vi "Get_camera_properties.vi"() -> ()   [LabVIEW 2012]
panel:
  in  "Camera Index":u32
  out "Function List":T1(array[cluster])
  out "error out":errorcluster
  out "Parameter Range":cluster{"min":dbl, "max":dbl, "step":dbl}
  out "Default parameter value":dbl
  out "Value Names":cluster{"Name":string, "Value":dbl}[](array[cluster])
  out "Parameter value":dbl
  in  "Parameter to query":u32(ring)=37 items=["BINNING"=1, "BITS PER CHANNEL"=2, "ACTIVE VIEW INDEX"=3, "CCD MODE"=4, "SENSOR MODE"=5, "READOUT MODE"=6, "EXPOSURE TIME"=7, "CONTRAST GAIN"=8, "CONTRAST OFFSET"=9, "LIGHT MODE"=10, "SENSITIVITY"=11, "WHITE BALANCE"=12, "PHOTON IMAGING MODE"=13, "HIGH DYNAMIC RANGE MODE"=14, "TRIGGER SOURCE"=15, "TRIGGER ACTIVE"=16, "TRIGGER MODE"=17, "TRIGGER POLARITY"=18, "TRIGGER GLOBAL EXPOSURE"=19, "FIRST TRIGGER BEHAVIOR"=20, "TRIGGER TIMES"=21, "OUTPUT TRIGGER POLARITY"=22, "OUTPUT TRIGGER DELAY"=23, "OUTPUT TRIGGER PERIOD"=24, "TEMPERATURE"=25, "TEMPERATURE TARGET"=26, "SENSOR COOLER FAN"=27, "MECHANICAL SHUTTER"=28, "BACK FOCUS POSITION"=29, "FRAMEBUNDLE MODE"=30, "FRAMEBUNDLE NUMBER"=31, "LINEBUNDLE HEIGHT"=32, "TRIGGER CONNECTOR"=33, "IMAGE PIXEL TYPE"=34, "OUTPUT TRIGGER KIND"=35, "READOUT DIRECTION"=36]
  out "Camera info":string
  in  "Info ID":u32(ring)=67109121 items=["BUS"=67109121, "CAMERA ID"=67109122, "VENDOR"=67109123, "MODEL"=67109124, "CAMERA VERSION"=67109125, "DRIVER VERSION"=67109126, "MODULE VERSIOIN"=67109127, "DCAMAPI VERSION"=67109128]
  in  "error in (no error)":errorcluster
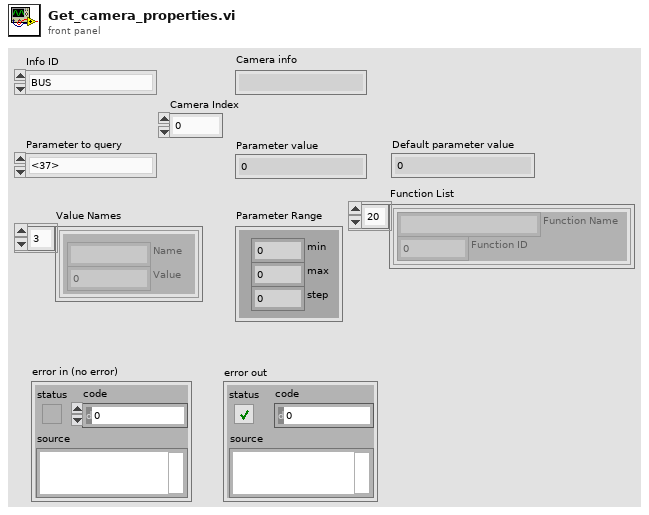
[diagram p1: front panel]
types:
  T1 = cluster{"Function Name":string, "Function ID":dbl}[]
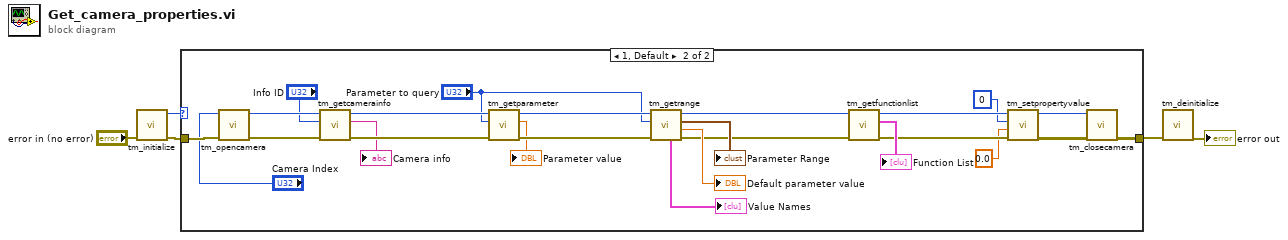
[diagram p0: block diagram]
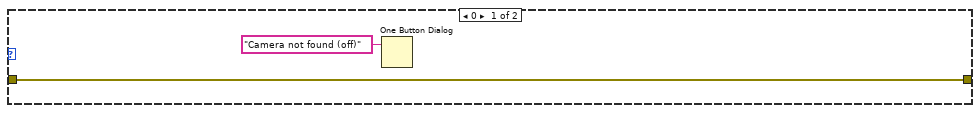
[diagram p2: hidden frame]
diagram:
  n1 = call <userlib>:"tm_initialize.vi"("error in (no error)"="error in (no error)") -> ("error out"=w5:errorcluster, "Number Of Cameras"=w3:u32)  [unwired: 9 in]
  n2 = case shown="1, Default" w3 {
    tunnel: w5 -> [w6 w32]
    tunnel: [w6 w17] -> w2
    frame 0 {
      n3 = One Button Dialog(message="Camera not found (off)") -> ()  [unwired: 1 in, 1 out]
    }
    frame 1, Default {
      n4 = call <userlib>:"tm_opencamera.vi"("error in (no error)"=w32, "Camera Index"="Camera Index") -> ("error out"=w31:errorcluster, "Handle out"=w27:u32)  [unwired: 8 in]
      n5 = call <userlib>:"tm_getcamerainfo.vi"("error in (no error)"=w31, "Info ID"="Info ID", "Handle in"=w27) -> ("error out"=w30:errorcluster, "String"=→"Camera info":string, "Handle out"=w26:u32)  [unwired: 6 in]
      n6 = call <userlib>:"tm_getparameter.vi"("error in (no error)"=w30, "Parameter"="Parameter to query", "Handle in"=w26) -> ("error out"=w29:errorcluster, "Value out"=→"Parameter value":dbl, "Handle out"=w25:u32)  [unwired: 6 in]
      n7 = call <userlib>:"tm_getrange.vi"("error in (no error)"=w29, "Parameter"="Parameter to query", "Handle in"=w25) -> ("error out"=w15:errorcluster, "default"=→"Default parameter value":dbl, "Range"=→"Parameter Range":cluster{"min":dbl, "max":dbl, "step":dbl}, "Handle out"=w16:u32, "Value Names"=→"Value Names":cluster{"Name":string, "Value":dbl}[])  [unwired: 2 in, 2 out]
      n8 = call <userlib>:"tm_getfunctionlist.vi"("error in (no error)"=w15, "Handle in"=w16) -> ("error out"=w13:errorcluster, "Function List"=→"Function List":T1, "Handle out"=w11:u32)  [unwired: 7 in]
      n9 = call <userlib>:"tm_setpropertyvalue.vi"("error in (no error)"=w13, "Value in"=sgl 0.0, "Property ID"=u32 0, "Handle in"=w11) -> ("error out"=w12:errorcluster, "Handle out"=w10:u32)  [unwired: 6 in]
      n10 = call <userlib>:"tm_closecamera.vi"("error in (no error)"=w12, "Handle in"=w10) -> ("error out"=w17:errorcluster)  [unwired: 9 in]
    }
  }
  n11 = call <userlib>:"tm_deinitialize.vi"("error in (no error)"=w2) -> ("error out"=→"error out":errorcluster)  [unwired: 10 in]
